vi "Create-Destroy.vi"(5 "Username":string, 6 "Password":string, 7 "Address":string, 8 "Error In":errorcluster) -> (0 "Error Out":errorcluster)   [LabVIEW 2017, in "Tests.lvlib" / "SFTP.lvlib"]
uses:
  SFTP.lvlib
  <vilib>/addons/_JKI Toolkits/Caraya/classes/Test/Test.lvclass
  <vilib>/addons/_JKI Toolkits/Caraya/classes/Assert/Assert.lvclass
  src/Toolkit/API/SFTP/SFTP.lvclass
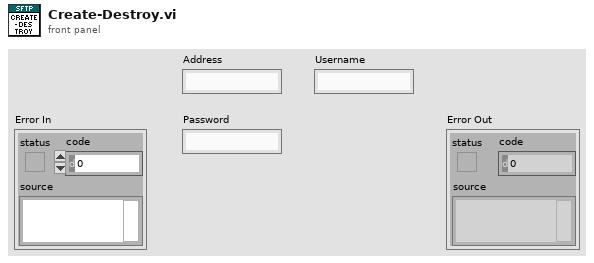
[diagram p1: front panel]
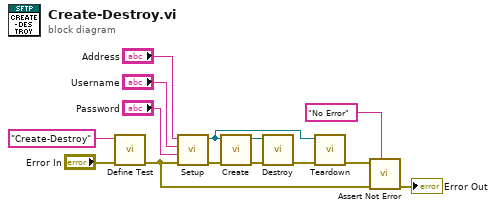
[diagram p0: block diagram]
diagram:
  n1 = call <vilib>:"Define Test.vi"("error in (no error)"="Error In", "Label (VI Title)"="Create-Destroy") -> ("error out"=w7:errorcluster)  [unwired: 9 in]
  n2 = call "Setup.vi"("Error In"=w7, "Password"="Password", "Username"="Username", "Address"="Address") -> ("Error Out"=w8:errorcluster, "Sesssion"=w3:refnum<class "Session.lvclass">)  [unwired: 6 in]
  n3 = call "Create.vi"("Error In"=w8, "Session"=w3) -> ("Error Out"=w9:errorcluster, "SFTP"=w10:refnum<class "SFTP.lvclass">)  [unwired: 8 in]
  n4 = call "Destroy.vi"("Error In"=w9, "SFTP"=w10) -> ("Error Out"=w2:errorcluster)  [unwired: 8 in, 1 out]
  n5 = call "Teardown.vi"("Error In"=w2, "Session"=w3) -> ("Error Out"=w1:errorcluster)  [unwired: 9 in]
  n6 = call <vilib>:"Assert Not Error.vi"("Label"="No Error", "error in (no error)"=w7, "Not Error?"=w1) -> ("error out"=→"Error Out":errorcluster)  [unwired: 8 in]
